vi "Add Series.vi"(10 "Series":refnum<class "Series.lvclass">, 11 "Result in":refnum<class "Result.lvclass">) -> (3 "Result out":refnum<class "Result.lvclass">)   [LabVIEW 2018, in "InfluxDB Client.lvlib" / "Result.lvclass"]
uses:
  Result.lvclass
  Series/Series.lvclass
  Result.lvclass/Result.ctl
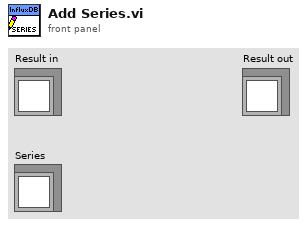
[diagram p1: front panel]
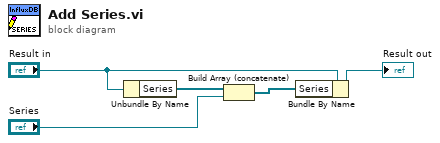
[diagram p0: block diagram]
diagram:
  n1 = Unbundle By Name("Result in") -> ("Series"=w3:refnum<class "Series.lvclass">[])
  n2 = Build Array (concatenate)(w3, "Series") -> (w1:refnum<class "Series.lvclass">[])
  n3 = Bundle By Name(cluster="Result in", "Series"=w1) -> (→"Result out":refnum<class "Result.lvclass">)
